vi "Analysis.Calc SPC from Meas Dim and Value Array.vi"(10 "Values_Str":string[](array[string]), 11 "Measurement Dimension":T1) -> (2 "SPC Data":string[](array[string]), 3 "Values":dbl[](array[numeric]))   [LabVIEW 2024]
uses:
  Analysis.Measurement Limit Info.ctl
  <vilib>/Analysis/NI_AALBase.lvlib
panel:
  out "ValueInCnt":i32
  out "ValueCnt":i32
  out "Values Sort":dbl[](array[numeric])
  # "Name, LL, UL, Min, Max, Mean, Stdev, Cpk"
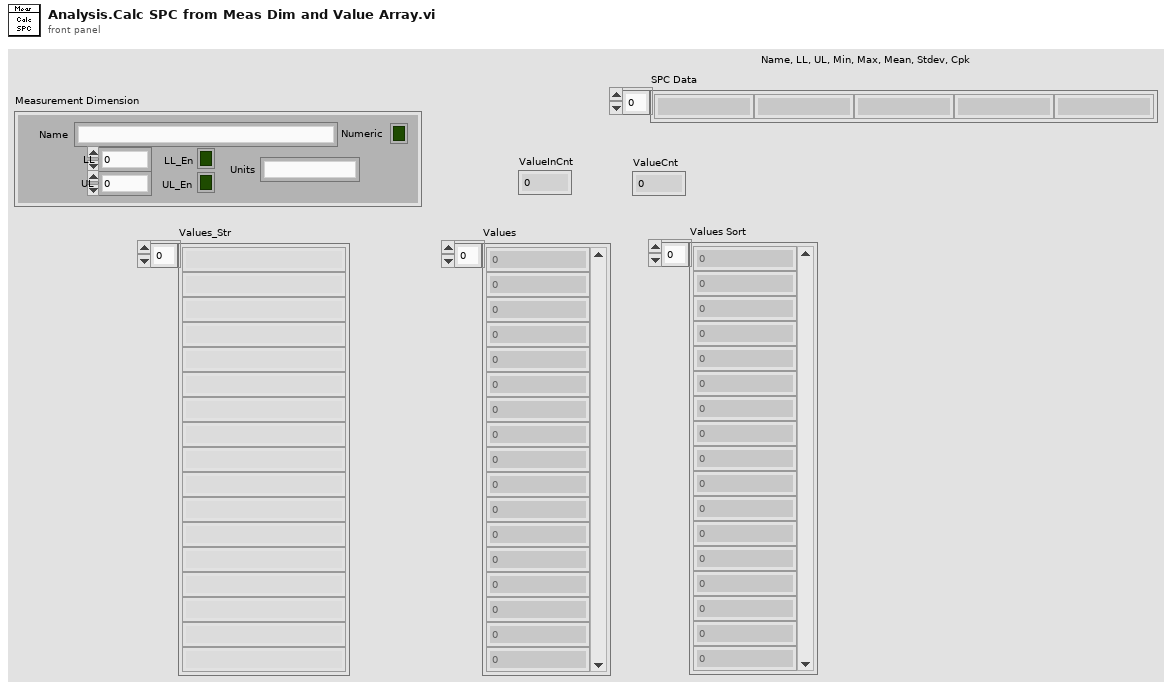
[diagram p1: front panel]
types:
  T1 = typedef "Analysis.Measurement Limit Info.ctl" = cluster{"Name":string, "Numeric":bool, "LL":dbl, "LL_En":bool, "UL":dbl, "UL_En":bool, "Units":string}
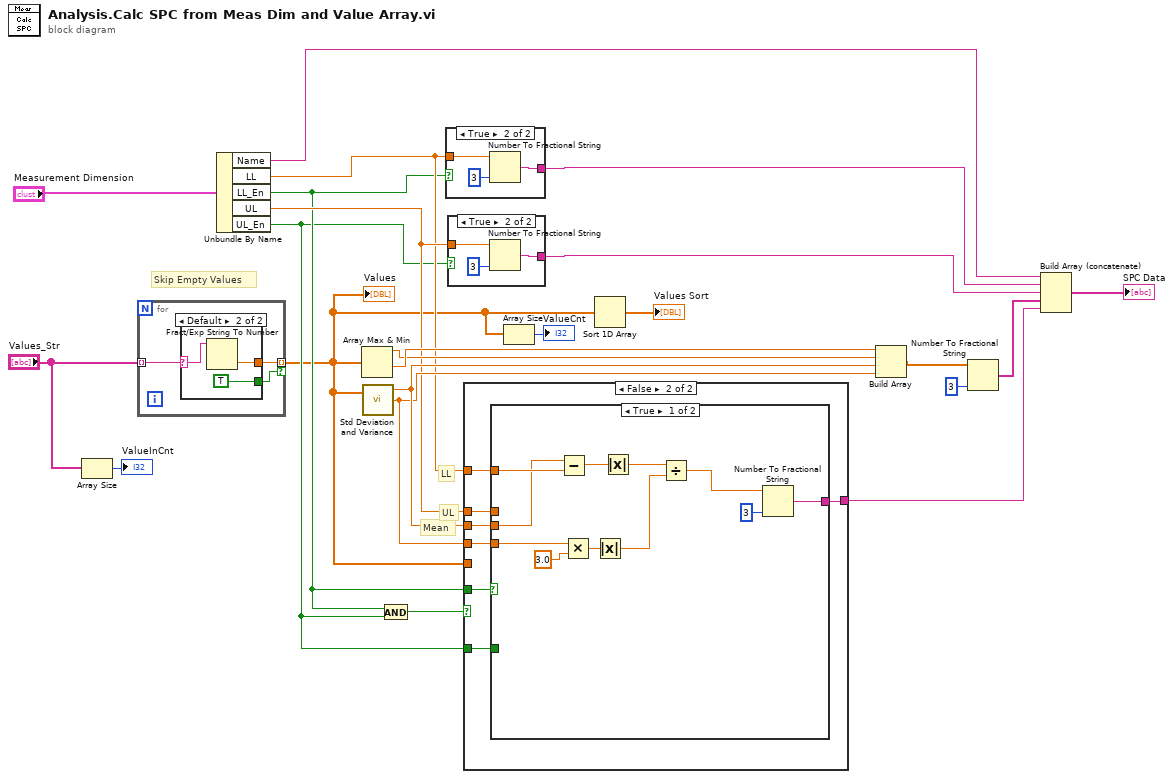
[diagram p0: block diagram]
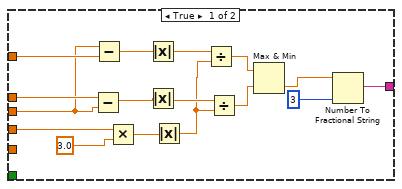
[diagram p2: hidden frame]
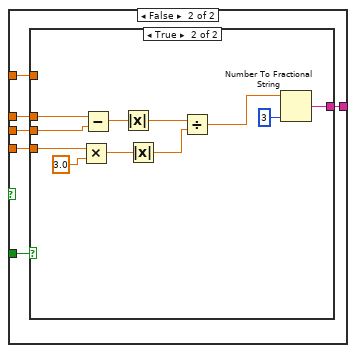
[diagram p3: hidden frame]
diagram:
  # "Skip Empty Values"
  # "UL"
  # "LL"
  # "Mean"
  n1 = Array Size(array="Values_Str") -> (size(s)=→"ValueInCnt":i32)
  n2 = for {
    tunnel: "Values_Str" -> [w26] mode=indexing
    tunnel: [w25] -> w4 mode=indexing if=w24
    n3 = case shown="Default" w26 {
      selector: w26 -> [_ w29]
      tunnel: [_ w28] -> w25
      tunnel: [_ TRUE] -> w24
      frame "" {
      }
      frame Default {
        n4 = Fract/Exp String To Number(string=w29) -> (number=w28:dbl)  [unwired: 3 in, 1 out]
      }
    }
  }
  "Values" <- w4
  n5 = Unbundle By Name("Measurement Dimension") -> ("Name"=w20:string, "LL"=w9:dbl, "LL_En"=w8:bool, "UL"=w10:dbl, "UL_En"=w7:bool)
  n6 = Array Max & Min(array=w4) -> (max value=w22:dbl, min value=w23:dbl)  [unwired: 2 out]
  n7 = call <vilib>:"Std Deviation and Variance.vi"("X"=w4) -> ("mean"=w13:dbl, "standard deviation"=w12:dbl)  [unwired: 1 in, 1 out]
  n8 = And(x=w8, y=w7) -> (x .and. y?=w11:bool)
  n9 = case shown="True" w8 {
    tunnel: [_ w32] -> w19
    tunnel: w9 -> [_ w31]
    frame False {
    }
    frame True {
      n10 = Number To Fractional String(number=w31, precision (6)=i16 3) -> (F-format string=w32:string)  [unwired: 2 in]
    }
  }
  n11 = case shown="True" w7 {
    tunnel: [_ w35] -> w18
    tunnel: w10 -> [_ w34]
    frame False {
    }
    frame True {
      n12 = Number To Fractional String(number=w34, precision (6)=i16 3) -> (F-format string=w35:string)  [unwired: 2 in]
    }
  }
  n13 = case shown="False" w11 {
    tunnel: w4 -> [_ _]
    tunnel: w13 -> [w47 w55]
    tunnel: w12 -> [w51 w58]
    tunnel: w10 -> [w49 w57]
    tunnel: w9 -> [w48 w56]
    tunnel: [w43 w53] -> w6
    tunnel: w8 -> [_ w54]
    tunnel: w7 -> [_ w52]
    frame True {
      n14 = Subtract(x=w49, y=w47) -> (x-y=w40:dbl)
      n15 = Subtract(x=w47, y=w48) -> (x-y=w41:dbl)
      n16 = Multiply(x=w51, y=3.0) -> (x*y=w37:dbl)
      n17 = Absolute Value(x=w41) -> (abs(x)=w38:dbl)
      n18 = Absolute Value(x=w40) -> (abs(x)=w39:dbl)
      n19 = Absolute Value(x=w37) -> (abs(x)=w36:dbl)
      n20 = Divide(x=w38, y=w36) -> (x/y=w46:dbl)
      n21 = Divide(x=w39, y=w36) -> (x/y=w45:dbl)
      n22 = Max & Min(x=w46, y=w45) -> (min(x,y)=w42:dbl)  [unwired: 1 out]
      n23 = Number To Fractional String(number=w42, precision (6)=i16 3) -> (F-format string=w43:string)  [unwired: 2 in]
    }
    frame False {
      n24 = case shown="True" w54 {
        tunnel: w58 -> [w69 w75]
        tunnel: w57 -> [_ w74]
        tunnel: w56 -> [w67 w73]
        tunnel: w55 -> [w66 w72]
        tunnel: [w64 w71] -> w53
        tunnel: w52 -> [_ w70]
        frame True {
          n25 = Subtract(x=w66, y=w67) -> (x-y=w62:dbl)
          n26 = Multiply(x=w69, y=3.0) -> (x*y=w60:dbl)
          n27 = Absolute Value(x=w60) -> (abs(x)=w59:dbl)
          n28 = Absolute Value(x=w62) -> (abs(x)=w61:dbl)
          n29 = Divide(x=w61, y=w59) -> (x/y=w63:dbl)
          n30 = Number To Fractional String(number=w63, precision (6)=i16 3) -> (F-format string=w64:string)  [unwired: 2 in]
        }
        frame False {
          n31 = case shown="True" w70 {
            tunnel: w75 -> [_ w86]
            tunnel: w74 -> [_ w84]
            tunnel: w73 -> [_ _]
            tunnel: w72 -> [_ w83]
            tunnel: [_ w81] -> w71
            frame False {
              # "N/A"
            }
            frame True {
              n32 = Multiply(x=w86, y=3.0) -> (x*y=w77:dbl)
              n33 = Subtract(x=w84, y=w83) -> (x-y=w79:dbl)
              n34 = Absolute Value(x=w79) -> (abs(x)=w78:dbl)
              n35 = Absolute Value(x=w77) -> (abs(x)=w76:dbl)
              n36 = Divide(x=w78, y=w76) -> (x/y=w80:dbl)
              n37 = Number To Fractional String(number=w80, precision (6)=i16 3) -> (F-format string=w81:string)  [unwired: 2 in]
            }
          }
        }
      }
    }
  }
  n38 = Array Size(array=w4) -> (size(s)=→"ValueCnt":i32)
  n39 = Sort 1D Array(array=w4) -> (sorted array=→"Values Sort":dbl[])
  n40 = Build Array(w23, w22, w13, w12) -> (w16:dbl[])
  n41 = Number To Fractional String(number=w16, precision (6)=i16 3) -> (F-format string=w15:string[])  [unwired: 2 in]
  n42 = Build Array (concatenate)(w20, w19, w18, w15, w6) -> (→"SPC Data":string[])
